vi "niScope Disable.vi"(0 "instrument handle":refnum<k15>, 11 "error in":errorcluster) -> (4 "instrument handle out":refnum<k15>, 15 "error out":errorcluster)   [LabVIEW 2011]
doc: "Aborts the current task, opens the data channel relays, and releases all RTSI and PFI lines. Use this VI for a condition where you want to stop the current acquisition and disable the channels."
uses:
  niScope_32.dll
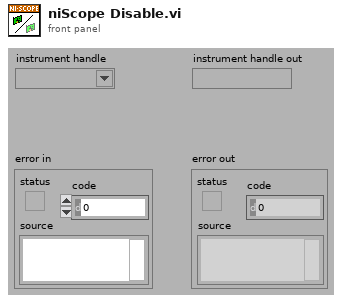
[diagram p1: front panel]
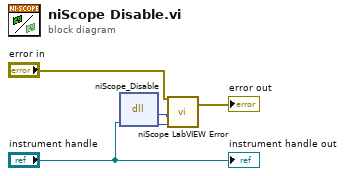
[diagram p0: block diagram]
diagram:
  n1 = dll-call lib="niScope_*.*" fn="niScope_Disable" ("niScope_reset")("instrumentHandle"="instrument handle") -> (w5:i32, "instrumentHandle"=w4:i32)  [unwired: 3 in, 2 out]
  n2 = call <instrlib>:"niScope LabVIEW Error.vi"("instrument handle"=w4, "niScope error code (0)"=w5, "error in (no error)"="error in") -> ("error out"=→"error out":errorcluster)  [unwired: 2 in]
  "instrument handle out" <- "instrument handle"
